vi "propsSI.vi"(4 "Second known var value [SI]":dbl, 5 "Second known var":string, 6 "First known var value [SI]":dbl, 7 "First known\nvar":string, 8 "error in (no error)":errorcluster, 9 "Fluid":string, 10 "module path":path, 11 "Desired var in":string) -> (0 "error out":errorcluster, 3 "Output [SI]":dbl)   [LabVIEW 2020]
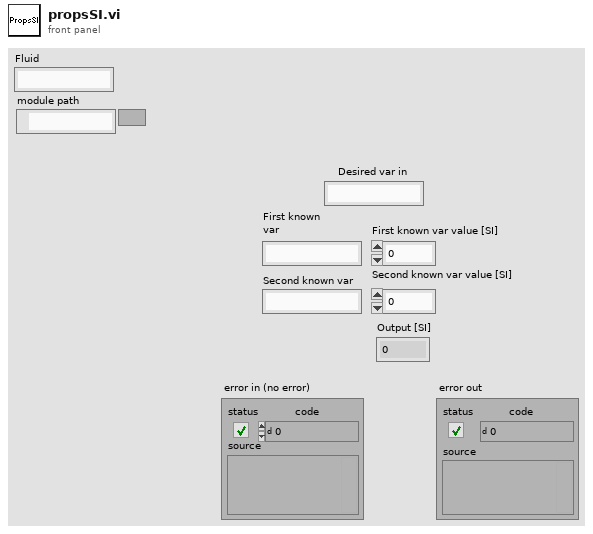
[diagram p1: front panel]
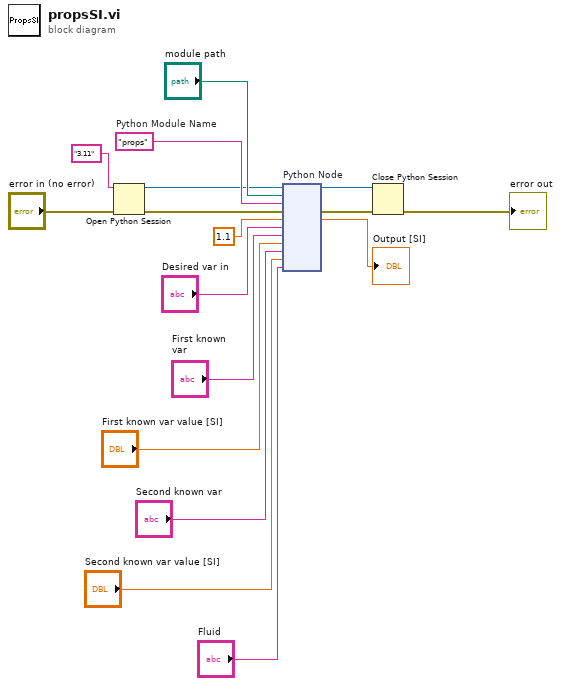
[diagram p0: block diagram]
diagram:
  w6 = "props"  # Python Module Name
  n1 = Open Python Session(python version="3.11", 3:"error in (no error)") -> (session out=w4:refnum<k35>, error out=w3:errorcluster)  [unwired: 1 in]
  n2 = node "Python Node"(w4, "module path", w6, w3, 1.1, "Desired var in", "First known\nvar", "First known var value [SI]", "Second known var", "Second known var value [SI]", "Fluid") -> (w5:refnum<k35>, w7:errorcluster, →"Output [SI]":dbl)  [unwired: 6 in, 2 out]
  n3 = Close Python Session(session in=w5, error in=w7) -> (11:→"error out":errorcluster)
